vi "Velocity.vi"(0 "connection ID":refnum<k5>, 3 "error in (no error)":errorcluster) -> (7 "connection ID out":refnum<k5>, 8 "Status":bool, 9 "Motor Status":string, 10 "error out":errorcluster)   [LabVIEW 2019]
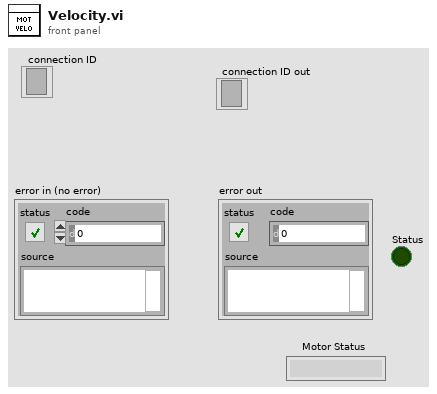
[diagram p1: front panel]
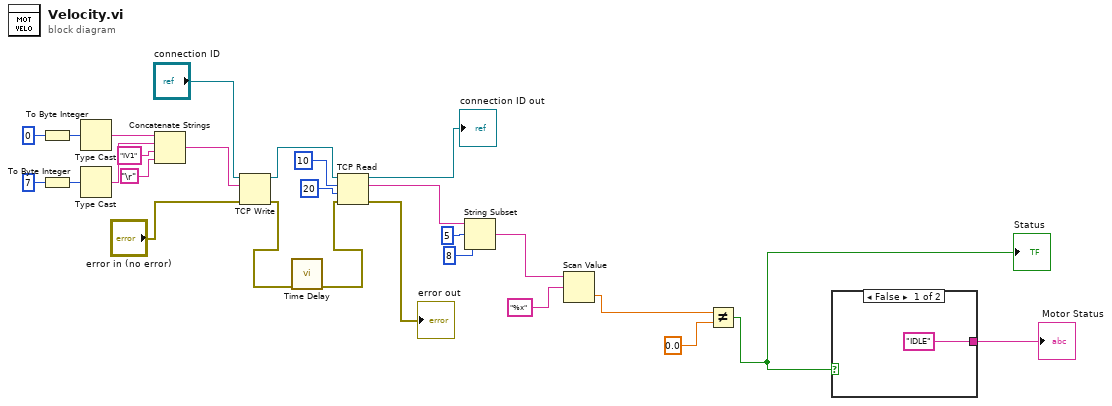
[diagram p0: block diagram]
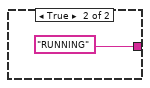
[diagram p2: hidden frame]
diagram:
  n1 = To Byte Integer(number=i8 0) -> (8bit integer=w26:i8)
  n2 = To Byte Integer(number=i8 7) -> (8bit integer=w27:i8)
  n3 = Type Cast(x=w26) -> (*(type *) &x=w20:string)  [unwired: 1 in]
  n4 = Type Cast(x=w27) -> (*(type *) &x=w21:string)  [unwired: 1 in]
  n5 = Concatenate Strings(w20, w21, "IV1" ("string"), "\r") -> (w23:string)
  n6 = TCP Write(connection ID="connection ID", data in=w23, error in (no error)="error in (no error)") -> (connection ID out=w16:refnum<k5>, error out=w14:errorcluster)  [unwired: 1 in, 1 out]
  n7 = call "Time Delay"("error in (no error)"=w14) -> ("error out"=w15:errorcluster)  [unwired: 10 in]
  n8 = TCP Read(connection ID=w16, bytes to read=10, error in (no error)=w15, 9:20 ("timeout ms (25000)")) -> (connection ID out=→"connection ID out":refnum<k5>, data out=w12:string, error out=→"error out":errorcluster)  [unwired: 1 in]
  n9 = String Subset(string=w12, offset (0)=5, length (rest)=8 ("length (rest)")) -> (substring=w1:string)
  n10 = Scan Value(string=w1, format string="%x") -> (value=w5:dbl)  [unwired: 1 in, 1 out]
  n11 = Not Equal?(x=w5, y=0.0) -> (x != y?=w3:bool)
  "Status" <- w3
  n12 = case shown="False" w3 {
    tunnel: ["IDLE" ("Motor") "RUNNING" ("Motor")] -> w2
    frame False {
    }
    frame True {
    }
  }
  "Motor Status" <- w2
